vi "Open_Close VI.vi"(8 "error in (no error)":errorcluster, 10 "NewVal":bool, 11 "VI in":refnum<vi>) -> (0 "error out":errorcluster)   [LabVIEW 2015]
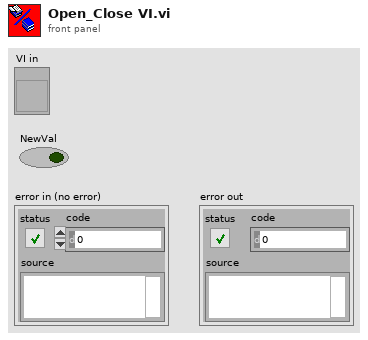
[diagram p1: front panel]
types:
  T1 = enum32{"Invalid", "Standard", "Closed", "Hidden", "Minimized", "Maximized"}
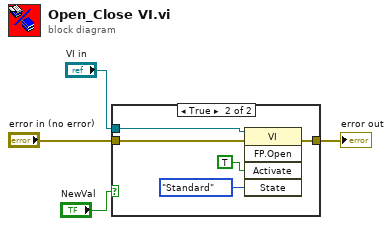
[diagram p0: block diagram]
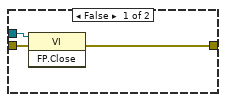
[diagram p2: hidden frame]
diagram:
  n1 = case shown="True" "NewVal" {
    tunnel: "VI in" -> [w7 w12]
    tunnel: "error in (no error)" -> [w5 w11]
    tunnel: [w6 w9] -> w1
    frame False {
      n2 = invoke class="VI" method="FP.Close"(reference=w7, error in=w5) -> (error out=w6:errorcluster)  [unwired: 1 in, 2 out]
    }
    frame True {
      n3 = invoke class="VI" method="FP.Open"(reference=w12, error in=w11, "Activate"=TRUE ("Activer ?"), "State"=T1."Standard") -> (error out=w9:errorcluster)  [unwired: 1 in, 4 out]
    }
  }
  "error out" <- w1
